vi "cmd-str-parser.vi"(6 "Enum":T1, 9 "name":string, 10 "value":string, 11 "command in":string) -> (1 "found?":bool, 2 "value out":string, 3 "command out":string)   [LabVIEW 2017]
uses:
  Control 1.ctl
panel:
  out "values":string[](array[string])
  out "names":string[](array[string])
  out "offset past match":i32
  # "command in/out is a string with a format:\n\"a=123,b=www,c=abc123\"\n\nuse the SET/GET menu to get or set variables in command in/out"
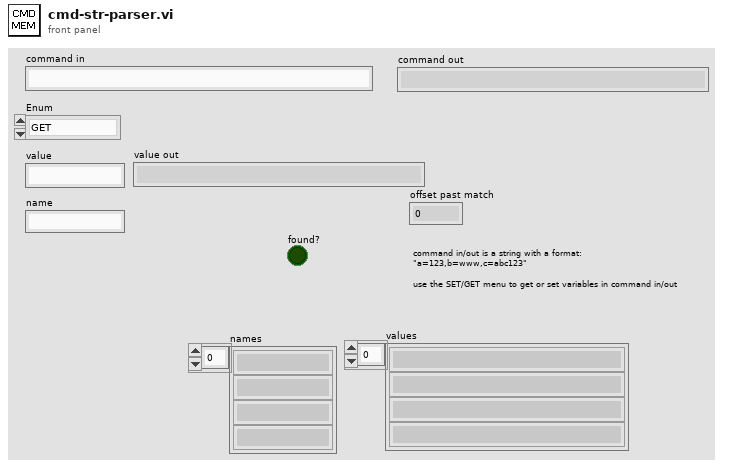
[diagram p1: front panel]
types:
  T1 = typedef "Control 1.ctl" = enum16{"GET", "SET", "DELETE", "INCREASE"}
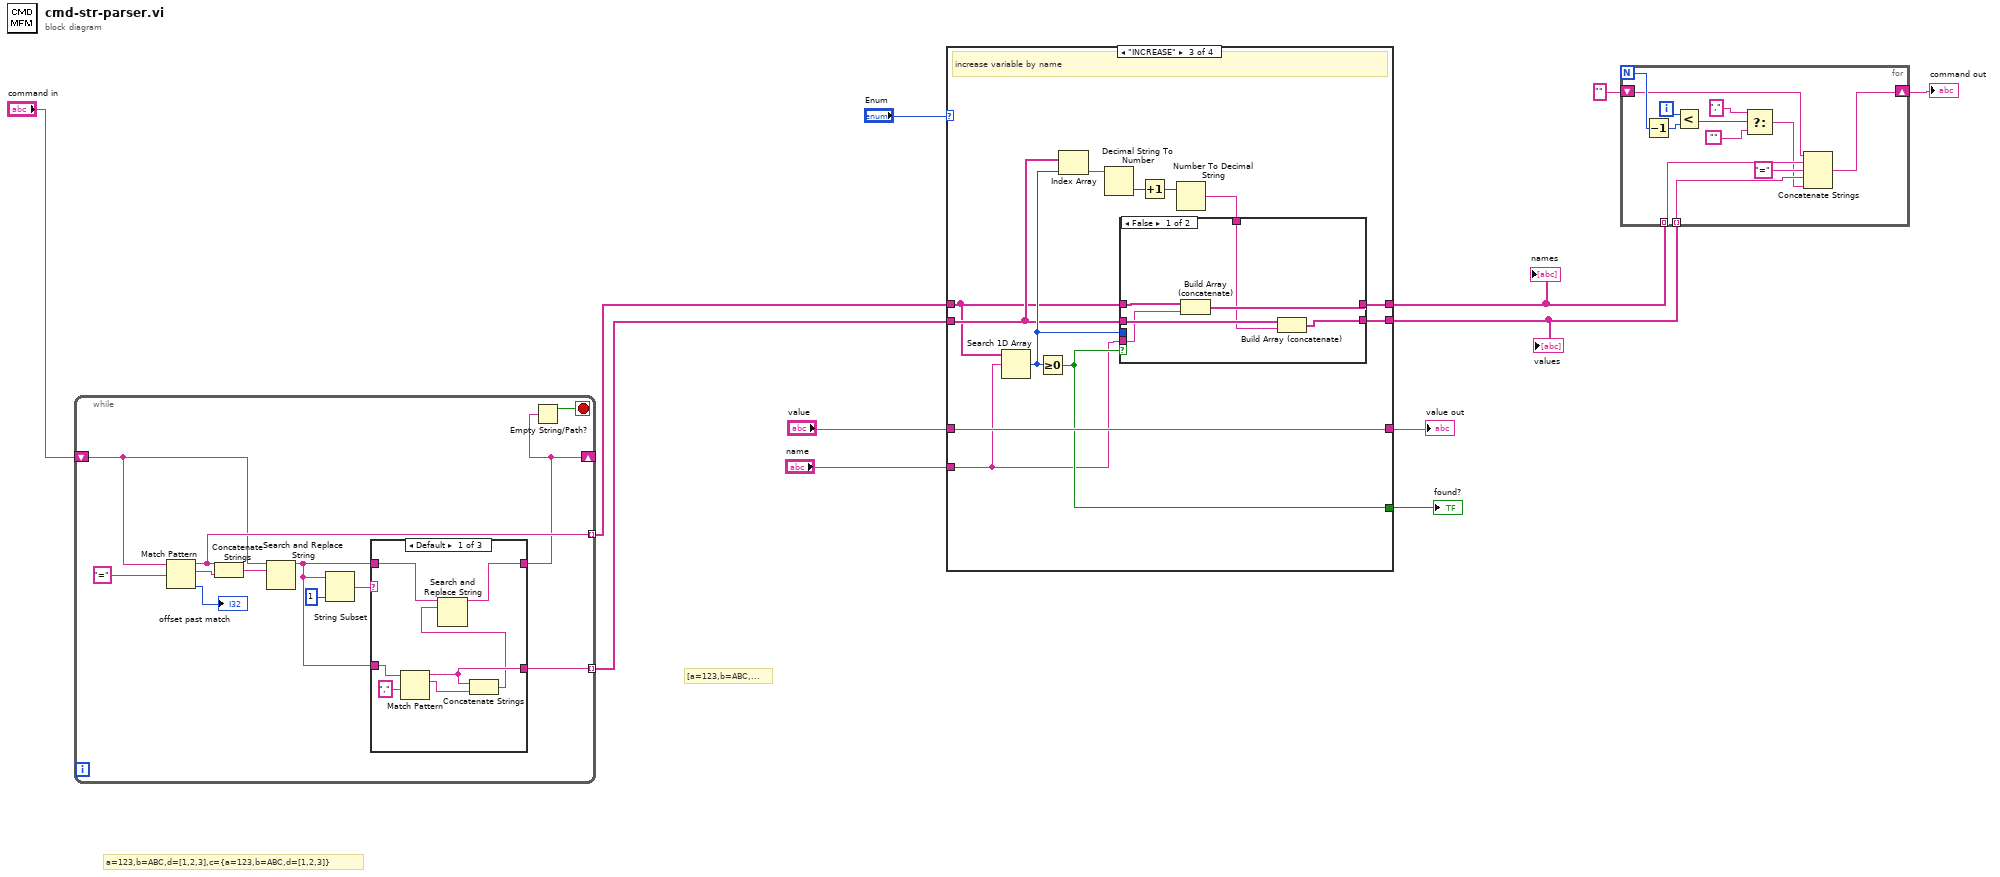
[diagram p0: block diagram]
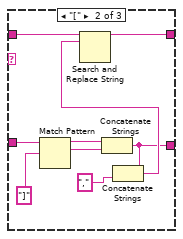
[diagram p2: hidden frame]
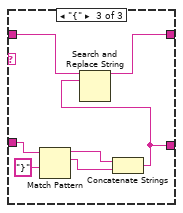
[diagram p3: hidden frame]
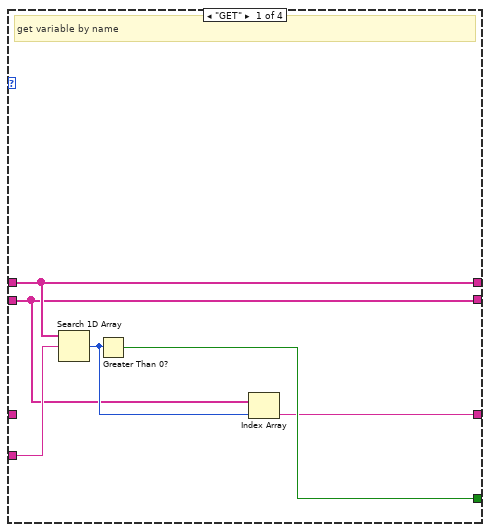
[diagram p4: hidden frame]
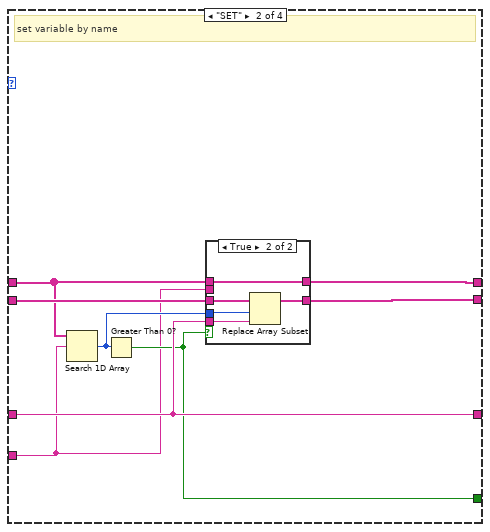
[diagram p5: hidden frame]
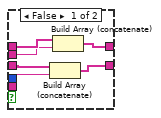
[diagram p6: hidden frame]
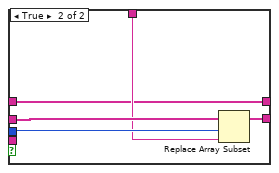
[diagram p7: hidden frame]
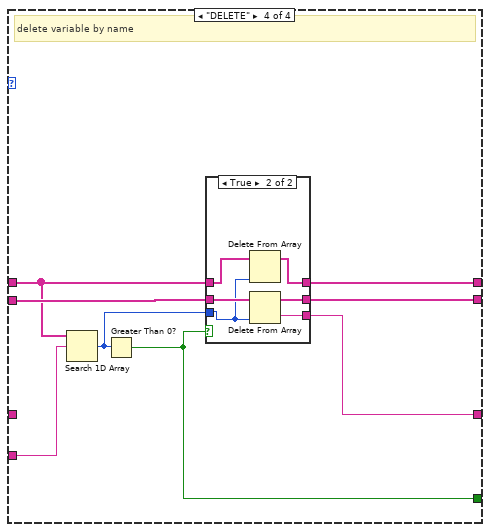
[diagram p8: hidden frame]
diagram:
  # "[a=123,b=ABC,..."
  # "a=123,b=ABC,d=[1,2,3],c={a=123,b=ABC,d=[1,2,3]}"
  n1 = while {
    shift-right: [w14] -> _
    shift-left: "command in" -> [w15]
    tunnel: [w17] -> w6 mode=indexing
    tunnel: [w16] -> w5 mode=indexing
    stop <- w23 stop-if-true
    n2 = Match Pattern(string=w15, regular expression="=") -> (before substring=w17:string, match substring=w22:string, offset past match=→"offset past match":i32)  [unwired: 1 in, 1 out]
    n3 = Concatenate Strings(w17, w22) -> (w20:string)
    n4 = Search and Replace String(input string=w15, search string=w20) -> (result string=w13:string)  [unwired: 6 in, 3 out]
    n5 = String Subset(string=w13, length (rest)=1 ("length (rest)")) -> (substring=w18:string)  [unwired: 1 in]
    n6 = case shown="Default" w18 {
      tunnel: w13 -> [w31 w40 w47]
      tunnel: [w27 w32 w41] -> w16
      tunnel: w13 -> [w29 w38 w45]
      tunnel: [w28 w37 w44] -> w14
      frame Default {
        n7 = Match Pattern(string=w31, regular expression=",") -> (before substring=w27:string, match substring=w26:string)  [unwired: 1 in, 2 out]
        n8 = Concatenate Strings(w27, w26) -> (w25:string)
        n9 = Search and Replace String(input string=w29, search string=w25) -> (result string=w28:string)  [unwired: 6 in, 3 out]
      }
      frame "[" {
        n10 = Match Pattern(string=w40, regular expression="]") -> (before substring=w34:string, match substring=w33:string)  [unwired: 1 in, 2 out]
        n11 = Concatenate Strings(w34, w33) -> (w32:string)
        n12 = Concatenate Strings(w32, "," ("string")) -> (w36:string)
        n13 = Search and Replace String(input string=w38, search string=w36) -> (result string=w37:string)  [unwired: 6 in, 3 out]
      }
      frame "{" {
        n14 = Match Pattern(string=w47, regular expression="}") -> (before substring=w43:string, match substring=w42:string)  [unwired: 1 in, 2 out]
        n15 = Concatenate Strings(w43, w42) -> (w41:string)
        n16 = Search and Replace String(input string=w45, search string=w41) -> (result string=w44:string)  [unwired: 6 in, 3 out]
      }
    }
    n17 = Empty String/Path?(string/path=w14) -> (empty?=w23:bool)
  }
  n18 = case shown="\"INCREASE\"" "Enum" {
    tunnel: "name" -> [w53 w54 w73 w103]
    tunnel: "value" -> [_ w61 w84 _]
    tunnel: [w49 w61 w84 w98] -> w9
    tunnel: w6 -> [w51 w55 w75 w97]
    tunnel: [w52 w59 w82 w101] -> w8
    tunnel: w5 -> [w48 w58 w81 w100]
    tunnel: [w51 w56 w74 w96] -> w4
    tunnel: [w48 w57 w80 w99] -> w3
    frame "GET" {
      # "get variable by name"
      n19 = Search 1D Array(1D array=w51, element=w53) -> (index of element=w50:i32)  [unwired: 1 in]
      n20 = Greater Than 0?(x=w50) -> (x > 0?=w52:bool)
      n21 = Index Array(array=w48, index=w50) -> (element=w49:string)
    }
    frame "SET" {
      # "set variable by name"
      n22 = Search 1D Array(1D array=w55, element=w54) -> (index of element=w60:i32)  [unwired: 1 in]
      n23 = Greater Than 0?(x=w60) -> (x > 0?=w59:bool)
      n24 = case shown="True" w59 {
        tunnel: w60 -> [_ w72]
        tunnel: w61 -> [w67 w71]
        tunnel: [w66 w70] -> w57
        tunnel: w58 -> [w65 w69]
        tunnel: w55 -> [w64 w68]
        tunnel: [w63 w68] -> w56
        tunnel: w54 -> [w62 _]
        frame False {
          n25 = Build Array (concatenate)(w65, w67) -> (w66:string[])
          n26 = Build Array (concatenate)(w64, w62) -> (w63:string[])
        }
        frame True {
          n27 = Replace Array Subset(array=w69, new element=w71, index=w72) -> (w70:string[])
        }
      }
    }
    frame "INCREASE" {
      # "increase variable by name"
      n28 = Search 1D Array(1D array=w75, element=w73) -> (index of element=w83:i32)  [unwired: 1 in]
      n29 = Greater Or Equal To 0?(x=w83) -> (x >= 0?=w82:bool)
      n30 = Index Array(array=w81, index=w83) -> (element=w77:string)
      n31 = Decimal String To Number(string=w77) -> (number=w79:i32)  [unwired: 2 in, 1 out]
      n32 = Increment(x=w79) -> (x+1=w78:i32)
      n33 = Number To Decimal String(number=w78) -> (decimal integer string=w76:string)  [unwired: 1 in]
      n34 = case shown="False" w82 {
        tunnel: w83 -> [_ w93]
        tunnel: [w86 w95] -> w80
        tunnel: w81 -> [w90 w94]
        tunnel: w76 -> [w87 w92]
        tunnel: [w88 w91] -> w74
        tunnel: w75 -> [w89 w91]
        tunnel: w73 -> [w85 _]
        frame False {
          n35 = Build Array (concatenate)(w89, w85) -> (w88:string[])
          n36 = Build Array (concatenate)(w90, w87) -> (w86:string[])
        }
        frame True {
          n37 = Replace Array Subset(array=w94, new element=w92, index=w93) -> (w95:string[])
        }
      }
    }
    frame "DELETE" {
      # "delete variable by name"
      n38 = Search 1D Array(1D array=w97, element=w103) -> (index of element=w102:i32)  [unwired: 1 in]
      n39 = Greater Than 0?(x=w102) -> (x > 0?=w101:bool)
      n40 = case shown="True" w101 {
        tunnel: w102 -> [_ w106]
        tunnel: [w105 w111] -> w99
        tunnel: w100 -> [w105 w110]
        tunnel: [_ w109] -> w98
        tunnel: w97 -> [w104 w108]
        tunnel: [w104 w107] -> w96
        frame False {
        }
        frame True {
          n41 = Delete From Array(array=w108, index=w106) -> (array with subset deleted=w107:string[])  [unwired: 1 in, 1 out]
          n42 = Delete From Array(array=w110, index=w106) -> (deleted portion=w109:string, array with subset deleted=w111:string[])  [unwired: 1 in]
        }
      }
    }
  }
  "value out" <- w9
  "found?" <- w8
  "names" <- w4
  "values" <- w3
  n43 = for {
    N -> [w119]
    tunnel: w4 -> [w123] mode=indexing
    tunnel: w3 -> [w121] mode=indexing
    shift-right: [w113] -> w1
    shift-left: "" ("string") -> [w112]
    i -> [w120]
    n44 = Decrement(x=w119) -> (x-1=w118:i32)
    n45 = Less?(x=w120, y=w118) -> (x < y?=w117:bool)
    n46 = Select(t="," ("string"), s=w117, f="") -> (s? t:f=w114:string)
    n47 = Concatenate Strings(w112, w123, "=" ("string"), w121, w114) -> (w113:string)
  }
  "command out" <- w1
